vi "proj_sprawdzenie.vi"(6 "Plansza":i32[][](array[numeric]), 7 "Selection Start":T1, 9 "Kolumna":i32, 10 "Wiersz":i32, 11 "Tabela interaktywna":refnum<vi>) -> (0 "Kolumna wychodzaca":i32, 1 "Wiersz wychodzacy":i32, 3 "Numeric":i32)   [LabVIEW 2020]
uses:
  <vilib>/Utility/miscctls.llb/LVRowAndColumnTypeDef.ctl
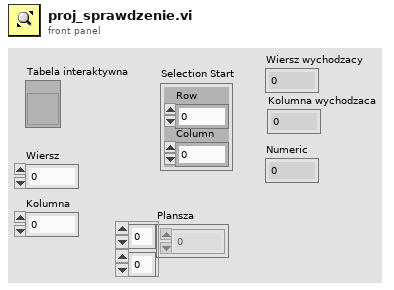
[diagram p1: front panel]
types:
  T1 = typedef "LVRowAndColumnTypeDef.ctl" = cluster{"Row":i32, "Column":i32}
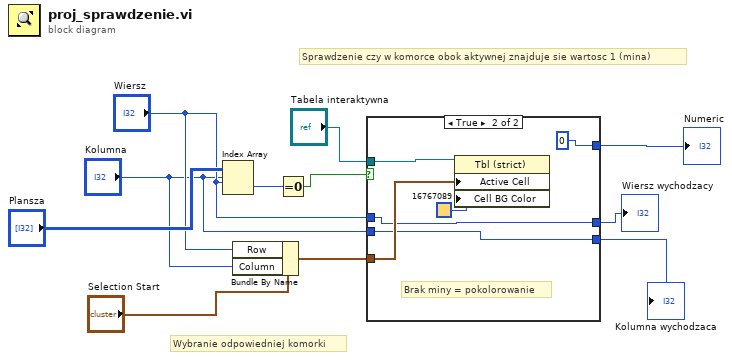
[diagram p0: block diagram]
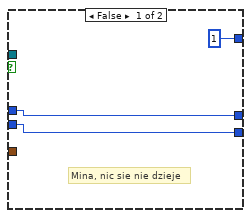
[diagram p2: hidden frame]
diagram:
  # "Wybranie odpowiedniej komorki"
  # "Sprawdzenie czy w komorce obok aktywnej znajduje sie wartosc 1 (mina)"
  n1 = Index Array(array="Plansza", index (row)="Wiersz", index (col)="Kolumna") -> (element=w8:i32)
  n2 = Bundle By Name(cluster="Selection Start", "Row"="Wiersz", "Column"="Kolumna") -> (w10:T1)
  n3 = Equal To 0?(x=w8) -> (x = 0?=w9:bool)
  n4 = case shown="True" w9 {
    tunnel: w10 -> [_ w20]
    tunnel: "Tabela interaktywna" -> [_ w18]
    tunnel: [1 0] -> w5
    tunnel: "Wiersz" -> [w13 w16]
    tunnel: "Kolumna" -> [w12 w15]
    tunnel: [w13 w16] -> w2
    tunnel: [w12 w15] -> w1
    frame False {
      # "Mina, nic sie nie dzieje"
    }
    frame True {
      # "Brak miny = pokolorowanie"
      n5 = property on="Property Node" class="Tbl (strict)"(reference=w18, "Active Cell"=w20, "Cell BG Color"=u32 16767089 ("Active Cell:Cell Background Color")) -> ()  [unwired: 1 in, 2 out]
    }
  }
  "Numeric" <- w5
  "Wiersz wychodzacy" <- w2
  "Kolumna wychodzaca" <- w1
